vi "Ex_Inst_Write LabVIEW Excel File.vi"(0 "Signals":dynamicdata(waveform), 1 "Reset":bool, 2 "Enable":bool=TRUE, 3 "Flush? (T)":bool=TRUE, 5 "error in (no error)":errorcluster, 8 "Filename":path, 11 "DAQmx Task":refnum<k21>) -> (16 "Filename Out":path, 17 "Saving Data":bool, 19 "error out":errorcluster)   [LabVIEW 2020]
doc: "Writes data to text-based measurement files (.lvm), binary measurement files (.tdm or .tdms), or Microsoft Excel files (.xlsx)."
uses:
  <vilib>/express/express shared/ExFile.llb/ex_FileFormats.ctl
  <vilib>/express/express shared/ExFile.llb/ex_userDefProperty.ctl
  <vilib>/express/express shared/ex_EditUserDefinedProperties/usiDataType.ctl
  <vilib>/express/express shared/ExFile.llb/ex_propertySource.ctl
  <vilib>/express/express output/ExFileWriteBlock.llb/ex_NewFileOptions.ctl
  <vilib>/express/express output/ExFileWriteBlock.llb/ex_ExcelAdvancedConfig.ctl
panel:
  in  "Live values":variant[](array[variant])
  in  "Comment":string
  in  "new_file":bool
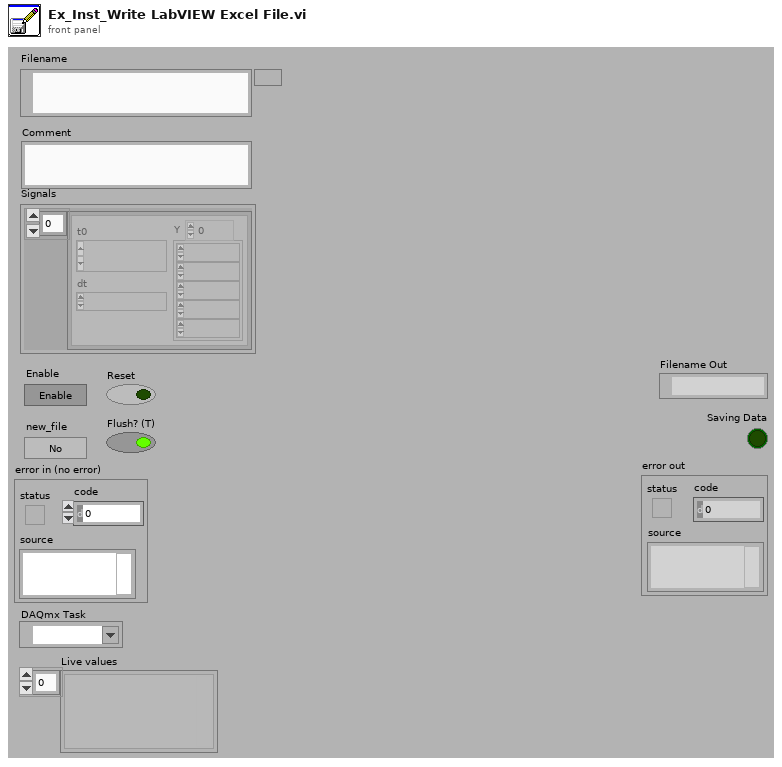
[diagram p1: front panel]
types:
  T1 = typedef "ex_FileFormats.ctl" = enum32{"lvm", "tdm", "tdms", "xlsx"}
  T2 = typedef "ex_userDefProperty.ctl" = cluster{"Name":string, "Object type":string, "usiDataType":T3, "propertySourceType":T4, "propertySource":string, "Value":variant, "ID":i32, "use def name":bool, "Source":string, "Built-in Prop":bool, "Attribute Type Enum":string[]}
  T3 = typedef "usiDataType.ctl" = enum16{"eNoTypeUsi", "eInt8Usi", "eInt16Usi", "eInt32Usi", "eInt64Usi", "eUInt8Usi", "eUInt16Usi", "eUInt32Usi", "eUInt64Usi", "eFloat32Usi", "eFloat64Usi", "- 0", "- 1", "- 2", "- 3", "- 4", "- 5", "- 6", "- 7", "- 8", "- 9", "eString8Usi", "eString16Usi", "eStringUsi", "eEnumUsi", "- 10", "- 11", "- 12", "- 13", "- 14", "eTimeUsi", "- 15", "- 16", "- 17", "- 18", "- 19", "- 20", "- 21", "- 22", "- 23", "eInstanceUsi", "eStoreUsi"}
  T4 = typedef "ex_propertySource.ctl" = enum16{"Manual", "System", "DAQmx Channel", "Terminal", "Ignore"}
  T5 = cluster{"Description":string, "Configure User Def Prop In":cluster{"user-def properties in":T2[], "selected nodes in":string[]}, "Comment":string, "DAQmx Task":string, "Live values":variant[]}
  T6 = cluster{"user-def properties in":T2[], "selected nodes in":string[]}
  T7 = cluster{"absolute time":bool, "Timestamp format":string}
  T8 = cluster{"new_file_mode":u16, "Width":i32, "time_format_string":string, "fixed_width":bool, "overwrite_mode_multi":i32, "serno_digits":i32}
  T9 = typedef "ex_NewFileOptions.ctl" = cluster{cluster{"new_file_iter":bool, "new_file_#iter":i32}, cluster{"new_file_samples":bool, "new_file_#samples":i32}, cluster{"new_file_size":bool, "new_file_max_size":i32}, cluster{"new_file_elaps_time":bool, "seconds":i32}, cluster{"new_file_daily":bool, "new_file_timeofday":i32}}
  T10 = typedef "ex_ExcelAdvancedConfig.ctl" = cluster{"absolute time":bool, "Timestamp format":string}
  T11 = cluster{"new_file":bool, "multi_file":bool, "Enable":bool, "File Dialog":bool, "x_columns":enum32{"none", "one", "multiple"}, "Ask each iteration":bool, "overwrite_mode":enum32{"overwrite", "overwrite & backup", "append", "next avail"}, "setting":cluster{"new_file_mode":u16, "Width":i32, "time_format_string":string, "fixed_width":bool, "overwrite_mode_multi":i32, "serno_digits":i32}, "new file options":T9, "reset":bool, "Flush":bool, "Static File Path in":path, "timestamp":T10}
  T12 = enum32{"overwrite", "overwrite & backup", "append", "next avail"}
  T13 = enum16{"overwrite", "overwrite & backup", "next avail"}
  T14 = cluster{"new_file_iter":bool, "new_file_#iter":i32}
  T15 = cluster{"new_file_samples":bool, "new_file_#samples":i32}
  T16 = cluster{"new_file_size":bool, "new_file_max_size":i32}
  T17 = cluster{"new_file_elaps_time":bool, "max_elapsed_seconds":i32}
  T18 = cluster{"new_file_daily":bool, "new_file_timeofday":i32}
  T19 = cluster{cluster{"new_file_iter":bool, "new_file_#iter":i32}, cluster{"new_file_samples":bool, "new_file_#samples":i32}, cluster{"new_file_size":bool, "new_file_max_size":i32}, cluster{"new_file_elaps_time":bool, "max_elapsed_seconds":i32}, cluster{"new_file_daily":bool, "new_file_timeofday":i32}}
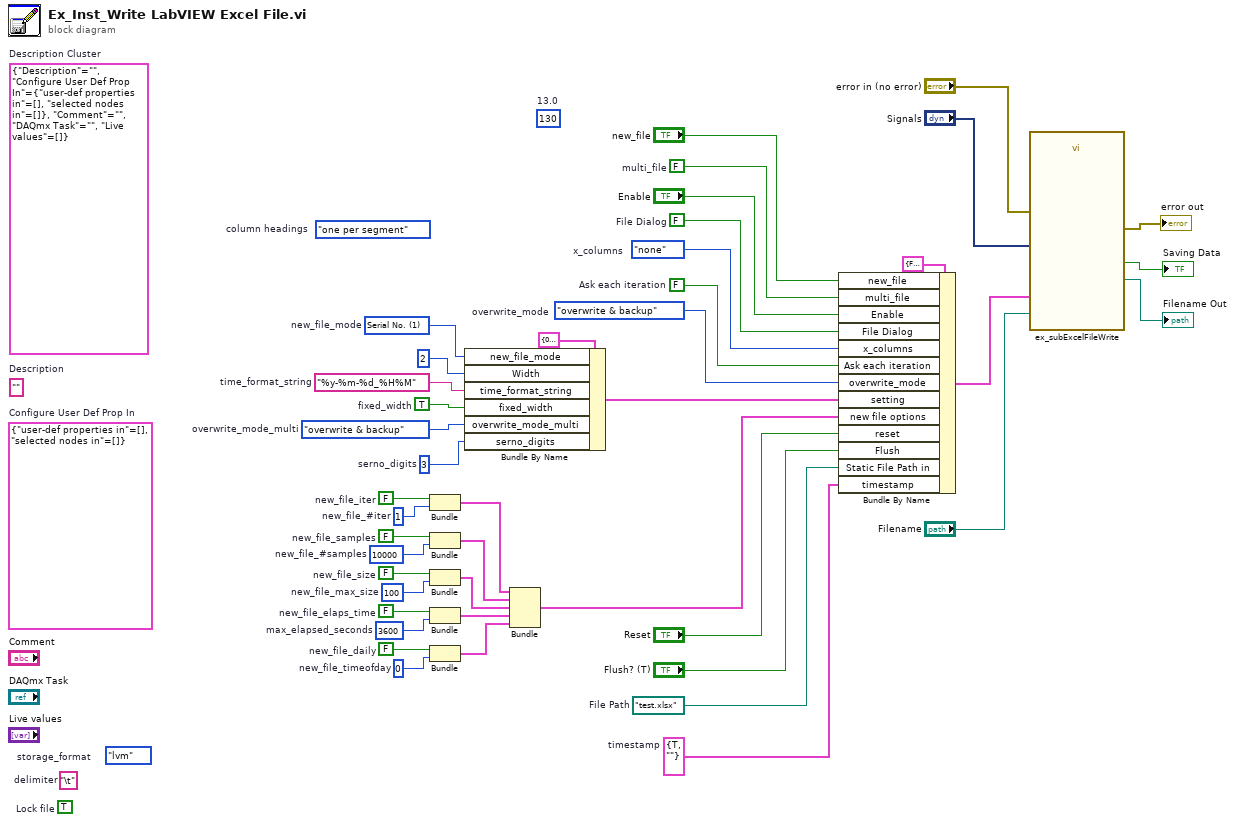
[diagram p0: block diagram]
diagram:
  (unwired) ex_FileFormats."lvm"  # storage_format
  (unwired) T5 {"Description"="", "Configure User Def Prop In"={"user-def properties in"=[], "selected nodes in"=[]}, "Comment"="", "DAQmx Task"="", "Live values"=[]}  # Description Cluster
  (unwired) TRUE  # Lock file
  (unwired) T6 {"user-def properties in"=[], "selected nodes in"=[]}  # Configure User Def Prop In
  (unwired) ""  # Description
  (unwired) "\t"  # delimiter
  w3 = T7 {"absolute time"=TRUE, "Timestamp format"=""}  # timestamp
  (unwired) 130  # 13.0
  w8 = T12."overwrite & backup"  # overwrite_mode
  w16 = enum32{"none", "one", "multiple"}."none"  # x_columns
  (unwired) enum32{"one per segment", "once", "none"}."one per segment"  # column headings
  w5 = FALSE  # Ask each iteration
  w13 = T13."overwrite & backup"  # overwrite_mode_multi
  w9 = u16 1 items=["Date & Time", "Serial No.", "Both"]  # new_file_mode
  w14 = "%y-%m-%d_%H%M"  # time_format_string
  w11 = TRUE  # fixed_width
  w12 = 3  # serno_digits
  w35 = 0  # new_file_timeofday
  w36 = FALSE  # new_file_daily
  w28 = 3600  # max_elapsed_seconds
  w37 = FALSE  # new_file_elaps_time
  w38 = 100  # new_file_max_size
  w39 = FALSE  # new_file_size
  w40 = 10000  # new_file_#samples
  w42 = 1  # new_file_#iter
  w41 = FALSE  # new_file_samples
  w43 = FALSE  # new_file_iter
  w18 = FALSE  # multi_file
  w1 = FALSE  # File Dialog
  w4 = path "test.xlsx"  # File Path
  n1 = Bundle("new_file_iter"=w43, "new_file_#iter"=w42) -> (w34:T14)  [unwired: 1 out]
  n2 = Bundle("new_file_samples"=w41, "new_file_#samples"=w40) -> (w33:T15)  [unwired: 1 out]
  n3 = Bundle("new_file_size"=w39, "new_file_max_size"=w38) -> (w30:T16)  [unwired: 1 out]
  n4 = Bundle("new_file_elaps_time"=w37, "max_elapsed_seconds"=w28) -> (w32:T17)  [unwired: 1 out]
  n5 = Bundle("new_file_daily"=w36, "new_file_timeofday"=w35) -> (w31:T18)  [unwired: 1 out]
  n6 = Bundle By Name(cluster=T8 {"new_file_mode"=0, "Width"=0, "time_format_string"="", "fixed_width"=FALSE, "overwrite_mode_multi"=0, "serno_digits"=0} ("setting"), "new_file_mode"=w9, "Width"=2, "time_format_string"=w14, "fixed_width"=w11, "overwrite_mode_multi"=w13, "serno_digits"=w12) -> (w7:T8)
  n7 = Bundle(w34, w33, w30, w32, w31) -> (w20:T19)  [unwired: 1 out]
  n8 = Bundle By Name(cluster=T11 {"new_file"=FALSE, "multi_file"=FALSE, "Enable"=TRUE, "File Dialog"=FALSE, "x_columns"=enum."none", "Ask each iteration"=FALSE, "overwrite_mode"=enum."overwrite", "setting"={"new_file_mode"=1, "Width"=2, "time_format_string"="%Y-%m-%d", "fixed_width"=TRUE, "overwrite_mode_multi"=1, "serno_digits"=3}, "new file options"={{"new_file_iter"=FALSE, "new_file_#iter"=0}, {"new_file_samples"=FALSE, "new_file_#samples"=0}, {"new_file_size"=FALSE, "new_file_max_size"=0}, {"new_file_elaps_time"=FALSE, "seconds"=0}, {"new_file_daily"=FALSE, "new_file_timeofday"=0}}, "reset"=FALSE, "Flush"=FALSE, "Static File Path in"=path "", "timestamp"={"absolute time"=TRUE, "Timestamp format"=""}} ("configurations"), "new_file"="new_file", "multi_file"=w18, "Enable"="Enable", "File Dialog"=w1, "x_columns"=w16, "Ask each iteration"=w5, "overwrite_mode"=w8, "setting"=w7, "new file options"=w20, "reset"="Reset", "Flush"="Flush? (T)", "Static File Path in"=w4, "timestamp"=w3) -> (w21:T11)
  n9 = call <vilib>:"ex_subExcelFileWrite.vi"("error in (no error)"="error in (no error)", "configurations"=w21, "File path"="Filename", "Signals"="Signals") -> ("error out"=→"error out":errorcluster, "Saving Data"=→"Saving Data":bool, "Filename out"=→"Filename Out":path)  [unwired: 5 in]
